vi "VISAControl.vi"(0 "VISA in":refnum<visa-resource-name>, 1 "IP":string, 2 "Mode":u32(ring) items=["Open", "Close", "Read", "Write", "Query"], 3 "Write Buffer":string="*IDN?", 4 "Name":string) -> (5 "VISA out":refnum<visa-resource-name>, 6 "Read Buffer":string)   [LabVIEW 2014]
uses:
  <vilib>/Instr/_visa.llb/VISA Open Access Mode.ctl
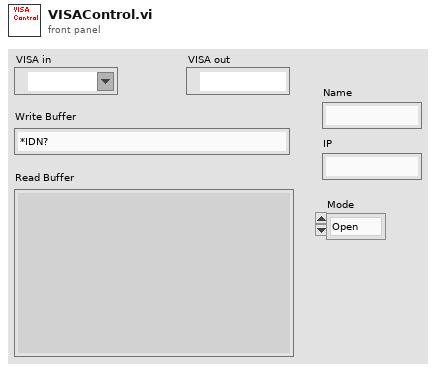
[diagram p1: front panel]
types:
  T1 = typedef "VISA Open Access Mode.ctl" = u32
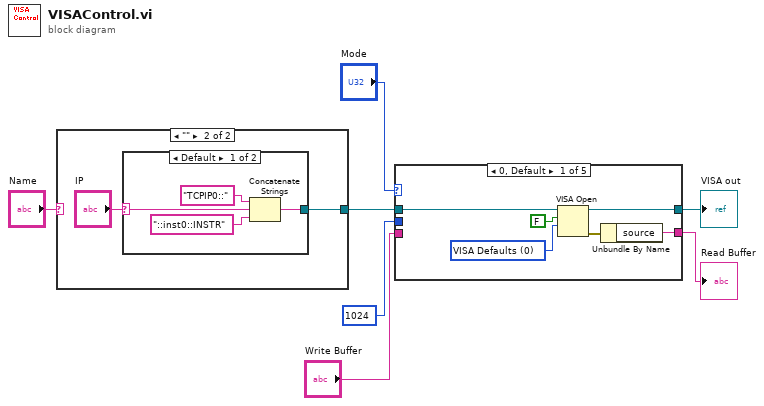
[diagram p0: block diagram]
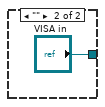
[diagram p3: hidden frame]
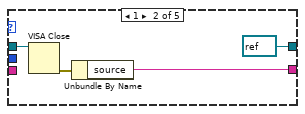
[diagram p4: hidden frame]
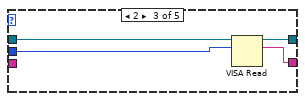
[diagram p5: hidden frame]
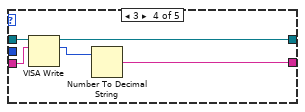
[diagram p6: hidden frame]
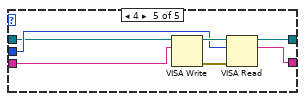
[diagram p7: hidden frame]
diagram:
  n1 = case shown="\"\"" "Name" {
    selector: "Name" -> [w8 _]
    tunnel: [w8 w9] -> w1
    frame Default {
    }
    frame "" {
      n2 = case shown="Default" "IP" {
        selector: "IP" -> [w12 _]
        tunnel: [w11 "VISA in"] -> w9
        frame Default {
          n3 = Concatenate Strings("TCPIP0::" ("string"), w12, "::inst0::INSTR" ("string")) -> (w11:string)
        }
        frame "" {
        }
      }
    }
  }
  n4 = case shown="0, Default" "Mode" {
    tunnel: [w18 refnum<visa-resource-name> refnum ("VISA resource name") w28 w34 w39] -> w3
    tunnel: "Write Buffer" -> [_ _ _ w33 w41]
    tunnel: [w16 w22 w29 w32 w38] -> w5
    tunnel: u32 1024 ("byte count") -> [_ _ w27 _ w37]
    tunnel: w1 -> [w19 w25 w26 w30 w35]
    frame 0, Default {
      w20 = T1 0 items=["VISA Defaults"=0, "Exclusive Lock"=1, "Load Configured Settings"=4] ("Access Mode")
      n5 = VISA Open(duplicate session (F)=FALSE, access mode=w20, VISA resource name=w19) -> (VISA resource name=w18:refnum<visa-resource-name>, error out=w17:errorcluster)  [unwired: 2 in]
      n6 = Unbundle By Name(w17) -> ("source"=w16:string)
    }
    frame 1 {
      n7 = VISA Close(VISA resource name=w25) -> (error out=w23:errorcluster)  [unwired: 1 in]
      n8 = Unbundle By Name(w23) -> ("source"=w22:string)
    }
    frame 2 {
      n9 = VISA Read(VISA resource name=w26, byte count=w27) -> (VISA resource name out=w28:refnum<visa-resource-name>, read buffer=w29:string)  [unwired: 1 in, 2 out]
    }
    frame 3 {
      n10 = VISA Write(VISA resource name=w30, write buffer=w33) -> (VISA resource name out=w34:refnum<visa-resource-name>, return count=w31:u32)  [unwired: 1 in, 1 out]
      n11 = Number To Decimal String(number=w31) -> (decimal integer string=w32:string)  [unwired: 1 in]
    }
    frame 4 {
      n12 = VISA Write(VISA resource name=w35, write buffer=w41) -> (VISA resource name out=w40:refnum<visa-resource-name>, error out=w36:errorcluster)  [unwired: 1 in, 1 out]
      n13 = VISA Read(VISA resource name=w40, byte count=w37, error in (no error)=w36) -> (VISA resource name out=w39:refnum<visa-resource-name>, read buffer=w38:string)  [unwired: 2 out]
    }
  }
  "Read Buffer" <- w5
  "VISA out" <- w3
